vi "u2pwm.vi"(2 "U":dbl[](array[numeric])) -> (14 "dc_u_t 0":dbl, 15 "dc_u_t 1":dbl, 16 "dc_u_t 2":dbl, 17 "dc_rotation_t 0":dbl, 18 "dc_rotation_t 1":dbl, 19 "dc_rotation_t 2":dbl)   [LabVIEW 2014]
uses:
  <vilib>/imath/engines/lvmath2/RunTimeEngine/NodeEndStatement/NIMS_NodeEndStatement_Output.vi
  <instcachedir>/0/NIMS_NodeEndStatement_Output_53EC0D466D134D7ABD903AC30B43404B.lvgen/NIMS_NodeEndStatement_Output_53EC0D466D134D7ABD903AC30B43404B_001.vi
  <vilib>/imath/engines/lvmath2/RunTimeEngine/ErrorHandling/NIMS_Finalize Error.vi
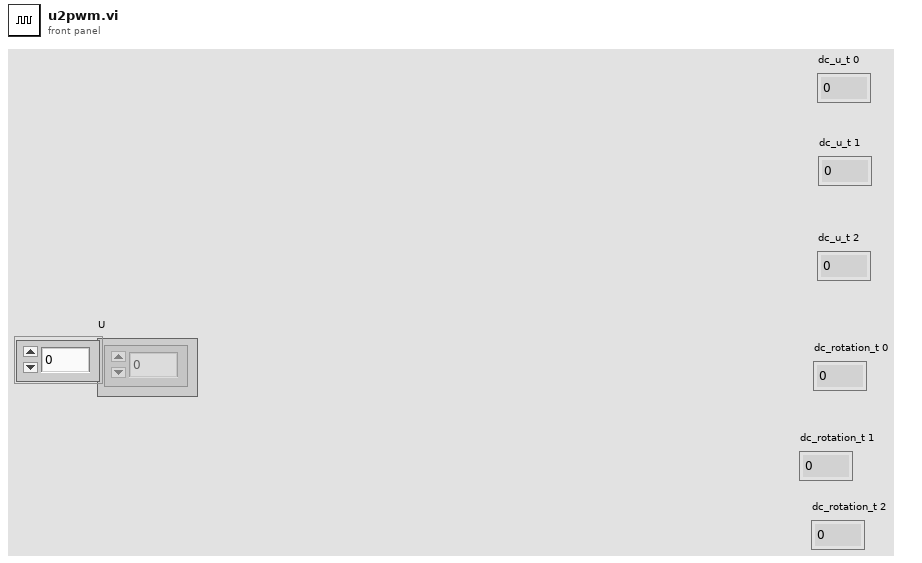
[diagram p1: front panel]
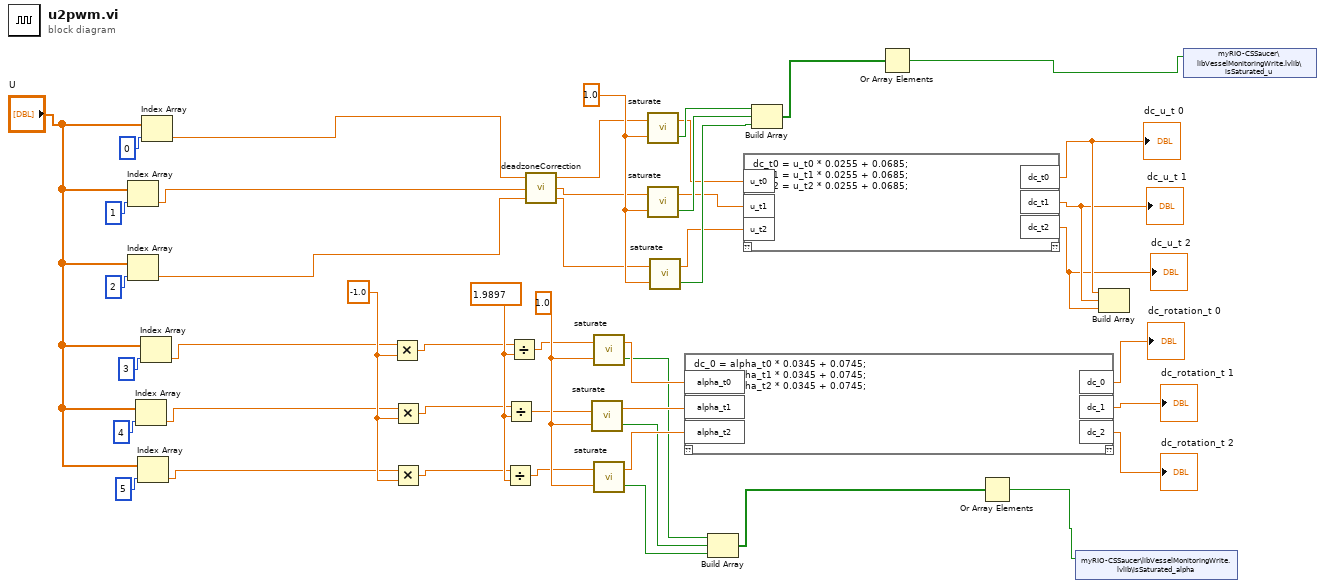
[diagram p0: block diagram]
diagram:
  w19 = -1.0
  w25 = 1.9897 ("y")
  w34 = 1.0 ("y")
  w44 = 1.0 ("amplitude")
  n1 = Index Array(array="U", index=1) -> (element=w6:dbl)
  n2 = Index Array(array="U", index=2) -> (element=w5:dbl)
  n3 = Index Array(array="U", index=4) -> (element=w3:dbl)
  n4 = Index Array(array="U", index=5) -> (element=w2:dbl)
  n5 = Index Array(array="U", index=3) -> (element=w4:dbl)
  n6 = Index Array(array="U", index=0) -> (element=w7:dbl)
  n7 = Multiply(x=w4, y=w19) -> (x*y=w22:dbl)
  n8 = Multiply(x=w3, y=w19) -> (x*y=w21:dbl)
  n9 = Multiply(x=w2, y=w19) -> (x*y=w20:dbl)
  n10 = Divide(x=w20, y=w25) -> (x/y=w23:dbl)
  n11 = Divide(x=w21, y=w25) -> (x/y=w24:dbl)
  n12 = Divide(x=w22, y=w25) -> (x/y=w26:dbl)
  n13 = call "deadzoneCorrection.vi"("u 2"=w5, "u 1"=w6, "u 0"=w7) -> ("out2"=w41:dbl, "out1"=w42:dbl, "out0"=w43:dbl)
  n14 = call "saturate.vi"("amplitude"=w34, "value"=w24) -> ("sat"=w28:bool, "saturated"=w32:dbl)
  n15 = call "saturate.vi"("amplitude"=w34, "value"=w26) -> ("sat"=w29:bool, "saturated"=w31:dbl)
  n16 = call "saturate.vi"("amplitude"=w34, "value"=w23) -> ("sat"=w27:bool, "saturated"=w33:dbl)
  n17 = call "saturate.vi"("amplitude"=w44, "value"=w43) -> ("sat"=w40:bool, "saturated"=w37:dbl)
  n18 = call "saturate.vi"("amplitude"=w44, "value"=w42) -> ("sat"=w39:bool, "saturated"=w36:dbl)
  n19 = call "saturate.vi"("amplitude"=w44, "value"=w41) -> ("sat"=w38:bool, "saturated"=w35:dbl)
  n20 = mathscript code="dc_0 = alpha_t0 * 0.0345 + 0.0745;\ndc_1 = alpha_t1 * 0.0345 + 0.0745;\ndc_2 = alpha_t2 * 0.0345 + 0.0745;"("alpha_t0"=w31, "alpha_t1"=w32, "alpha_t2"=w33) -> ("dc_0"=→"dc_rotation_t 0":dbl, "dc_1"=→"dc_rotation_t 1":dbl, "dc_2"=→"dc_rotation_t 2":dbl)  [unwired: 1 in, 1 out]
  n21 = Build Array(w29, w28, w27) -> (w30:bool[])
  n22 = mathscript code="dc_t0 = u_t0 * 0.0255 + 0.0685;\ndc_t1 = u_t1 * 0.0255 + 0.0685;\ndc_t2 = u_t2 * 0.0255 + 0.0685;"("u_t0"=w37, "u_t1"=w36, "u_t2"=w35) -> ("dc_t0"=w18:dbl, "dc_t1"=w17:dbl, "dc_t2"=w16:dbl)  [unwired: 1 in, 1 out]
  "dc_u_t 0" <- w18
  "dc_u_t 1" <- w17
  "dc_u_t 2" <- w16
  n23 = Build Array(w40, w39, w38) -> (w45:bool[])
  n24 = Or Array Elements(Boolean array=w45) -> (logical OR=w14:bool)
  n25 = Or Array Elements(Boolean array=w30) -> (logical OR=w15:bool)
  n26 = shared-variable "myRIO-CSSaucer\\libVesselMonitoringWrite.lvlib\\isSaturated_alpha"(w15) -> ()  [unwired: 1 in, 1 out]
  n27 = Build Array(w18, w17, w16) -> ()  [unwired: 1 out]
  n28 = shared-variable "myRIO-CSSaucer\\libVesselMonitoringWrite.lvlib\\isSaturated_u"(w14) -> ()  [unwired: 1 in, 1 out]
